vi "AlazarDSPGetNextBufferU16.vi"(4 "error in (no error)":errorcluster, 5 "timeout_ms":u32, 6 "Buffer":u16[](array[numeric]), 7 "Handle":u64) -> (0 "error out":errorcluster, 1 "Return Code":u32, 2 "Buffer":u16[](array[numeric]), 3 "Handle":u64)   [LabVIEW 2009]
doc: "This function returns when the board has received sufficient trigger events to fill the buffer, or the timeout interval has elapsed. To use this function, AlazarBeforeAsyncRead must be called with the ADMA_ALLOC_BUFFERS flag."
uses:
  ATSApi.dll
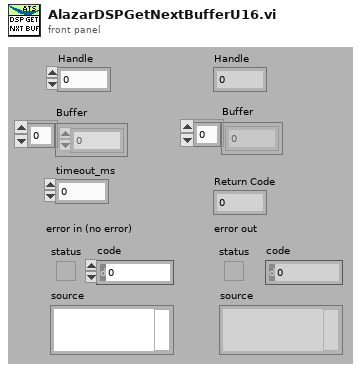
[diagram p1: front panel]
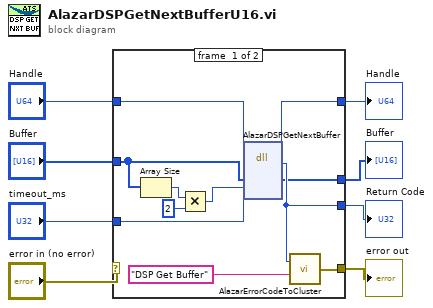
[diagram p0: block diagram]
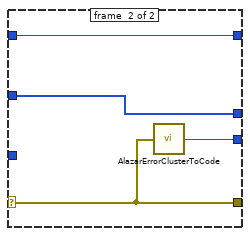
[diagram p2: hidden frame]
diagram:
  n1 = case shown="No Error" "error in (no error)" {
    selector: "error in (no error)" -> [_ w23]
    tunnel: [w16 w23] -> w7
    tunnel: [w18 w22] -> w6
    tunnel: "Handle" -> [w19 w21]
    tunnel: [w15 w21] -> w4
    tunnel: "Buffer" -> [w12 w20]
    tunnel: "timeout_ms" -> [w13 _]
    tunnel: [w14 w20] -> w1
    frame #0 {
      n2 = Array Size(array=w12) -> (size(s)=w11:i32)
      n3 = Multiply(x=w11, y=2) -> (x*y=w9:i32)
      n4 = dll-call lib="ATSApi.dll" fn="AlazarDSPGetNextBuffer"("handle"=w19, "buffer"=w12, "bytesToCopy"=w9, "timeout_ms"=w13) -> ("return type"=w18:u32, "handle"=w15:u64, "buffer"=w14:u16[])  [unwired: 5 in, 2 out]
      n5 = call "AlazarErrorCodeToCluster.vi"("Message"="DSP Get Buffer", "Error Code"=w18) -> ("error out"=w16:errorcluster)
    }
    frame #1 {
      n6 = call "AlazarErrorClusterToCode.vi"("error in (no error)"=w23) -> ("Error Code"=w22:u32)
    }
  }
  "Handle" <- w4
  "error out" <- w7
  "Return Code" <- w6
  "Buffer" <- w1
